vi "Stage Polling Loop.vi"(11 "Stage Actor.lvlib:Stage.lvclass":refnum<class "Stage.lvclass">) -> ()   [LabVIEW 2018, in "Stage Actor.lvlib" / "Stage.lvclass"]
uses:
  Stage.lvclass
  C:/Program Files/National Instruments/LabVIEW 2018/vi.lib/MGI/Panel Manager/Panel Actor/Panel Actor/Panel Actor.lvclass
  <vilib>/ActorFramework/Message Enqueuer/Message Enqueuer.lvclass/Message Enqueuer.ctl
  <vilib>/ActorFramework/Message Enqueuer/Enqueue.vi
  Stage Messages/Read Position Msg/Read Position Msg.lvclass
  C:/Program Files/National Instruments/LabVIEW 2018/vi.lib/ActorFramework/Message/Message.lvclass
  Stage Messages/Read Digital Outputs Msg/Read Digital Outputs Msg.lvclass
  <vilib>/ActorFramework/Message Priority Queue/Priority Enqueue.vi
  <vilib>/MGI/Panel Manager/Panel Actor/Panel Actor/Panel Actor.lvclass
panel:
  in  "Stop":bool=TRUE
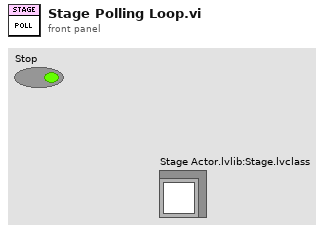
[diagram p1: front panel]
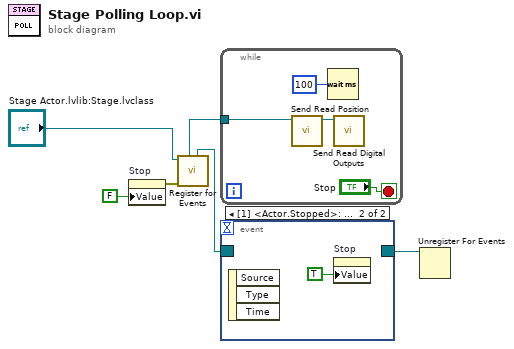
[diagram p0: block diagram]
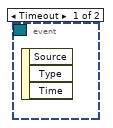
[diagram p2: hidden frame]
diagram:
  n1 = property on="Stop" class="Bool (strict)"("Value"=FALSE ("Stop")) -> (error out=w2:errorcluster)  [unwired: 2 in, 1 out]
  n2 = call <vilib>:"Register for Events.vi"("Error In"=w2, "Panel Actor in"="Stage Actor.lvlib:Stage.lvclass") -> ("Pnl Actor"=w5:refnum<event-registration>, "Self Enqueuer"=w1:refnum<class "Message Enqueuer.lvclass">)  [unwired: 6 in, 2 out]
  n3 = while {
    tunnel: w1 -> [w8]
    stop <- "Stop" stop-if-true
    n4 = call "Send Read Position.vi"("Message Enqueuer in"=w8) -> ("Message Enqueuer out"=w7:refnum<class "Message Enqueuer.lvclass">)  [unwired: 9 in, 1 out]
    n5 = Wait (ms)(milliseconds to wait=u32 100) -> ()  [unwired: 1 out]
    n6 = call "Send Read Digital Outputs.vi"("Message Enqueuer in"=w7) -> ()  [unwired: 9 in, 2 out]
  }
  n7 = event shown="[1] <Actor.Stopped>: User Event" {
    selector: w5 -> [_ _]
    dyn-events: [_ _] -> w4
    timeout: _ -> [_ _]
    event Timeout {
      n8 = event-data() -> ()  [unwired: 1 in, 3 out]
    }
    event User Event {
      n9 = event-data() -> ()  [unwired: 1 in, 3 out]
      n10 = property on="Stop" class="Bool (strict)"("Value"=TRUE ("Stop")) -> ()  [unwired: 2 in, 2 out]
    }
  }
  n11 = Unregister For Events(event registration refnum=w4) -> ()  [unwired: 1 in, 1 out]
